vi "Conversion_subVI.vi"(10 "Acceleration Unit in":bool, 11 "data":dbl) -> (3 "Numeric":dbl)   [LabVIEW 2023]
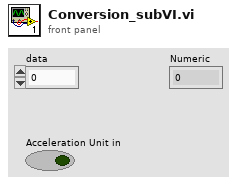
[diagram p1: front panel]
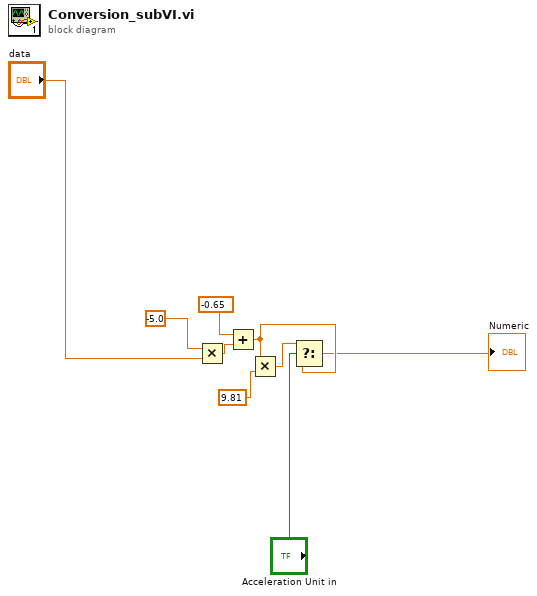
[diagram p0: block diagram]
diagram:
  n1 = Multiply(x=-5.0, y="data") -> (x*y=w2:dbl)
  n2 = Add(x=-0.65, y=w2) -> (x+y=w9:dbl)
  n3 = Multiply(x=w9, y=9.81) -> (x*y=w8:dbl)
  n4 = Select(t=w8, s="Acceleration Unit in", f=w9) -> (s? t:f=→"Numeric":dbl)
